vi "Get Joystick Type.vi"() -> (3 "Joystick Type":bool)   [LabVIEW 2014]
doc: "Returns the joystick type being used on the drive station computer."
uses:
  <vilib>/Rock Robotics/Network Tables/SD Read Boolean.vi
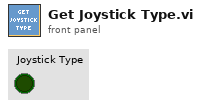
[diagram p1: front panel]
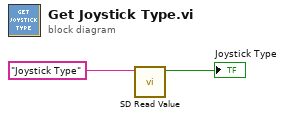
[diagram p0: block diagram]
diagram:
  n1 = call-poly <vilib>:"SD Read Value.vi"("Name"="Joystick Type") -> ("Boolean"=→"Joystick Type":bool)  [unwired: 8 in, 2 out]
